vi "send data.vi"() -> ()   [LabVIEW 2016]
uses:
  <vilib>/Instr/_visa.llb/Select Event Type.ctl
  <vilib>/Utility/error.llb/DialogType.ctl
  <vilib>/httpClient/LabVIEWHTTPClient.lvlib
panel:
  in  "Tab Control":enum32{"Page 1", "Page 2"}(tab)
  out "Voltage in range?":bool
  out "Amperage in range?":bool
  out "Pressure in range?":bool
  out "Temperature in range?":bool
  out "Current values":cluster{dbl, dbl, dbl, dbl}(graph)
  in  "VISA resource name":refnum<visa-resource-name>
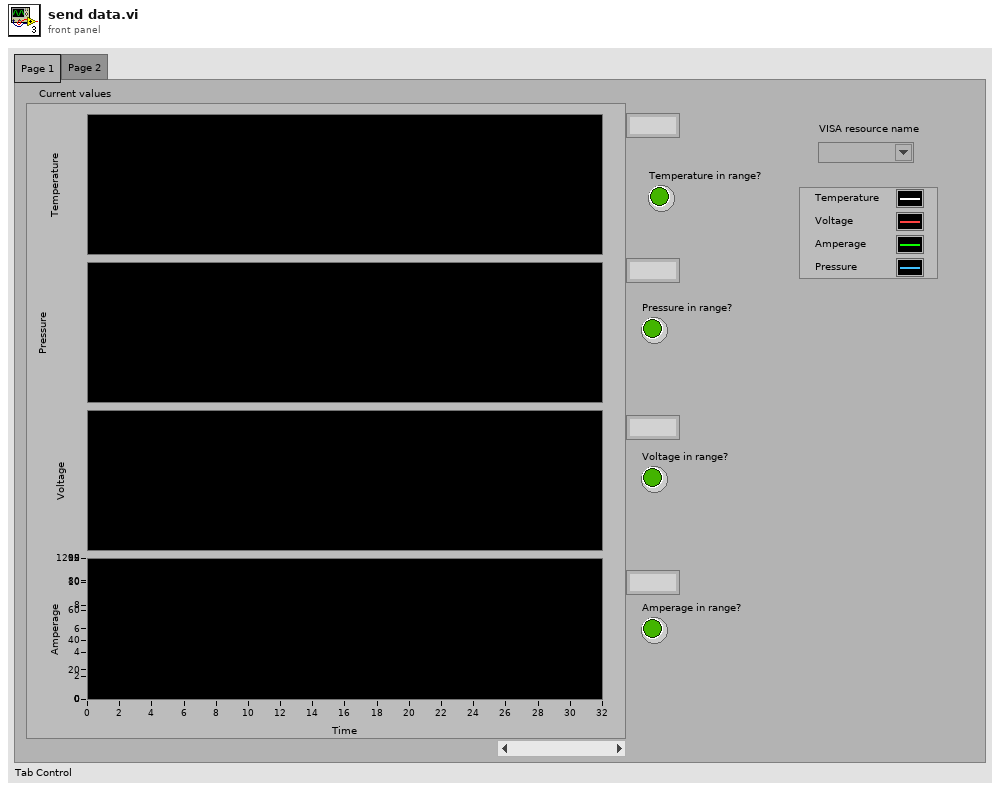
[diagram p1: front panel]
types:
  T1 = typedef "DialogType.ctl" = u16
  T2 = typedef "Select Event Type.ctl" = u32
  T3 = typedef "LabVIEWHTTPClient.lvlib/ClientHandle.ctl" = refnum<k1>
  T4 = cluster{"queue out":refnum<queue>, "queue out":refnum<queue>, "queue out":refnum<queue>, "queue out":refnum<queue>, "queue out":refnum<queue>}
  T5 = cluster{"DS18B20 value":dbl, "BMP180 value":dbl, " potentiometer value":dbl, "ACS712-30A value":dbl}
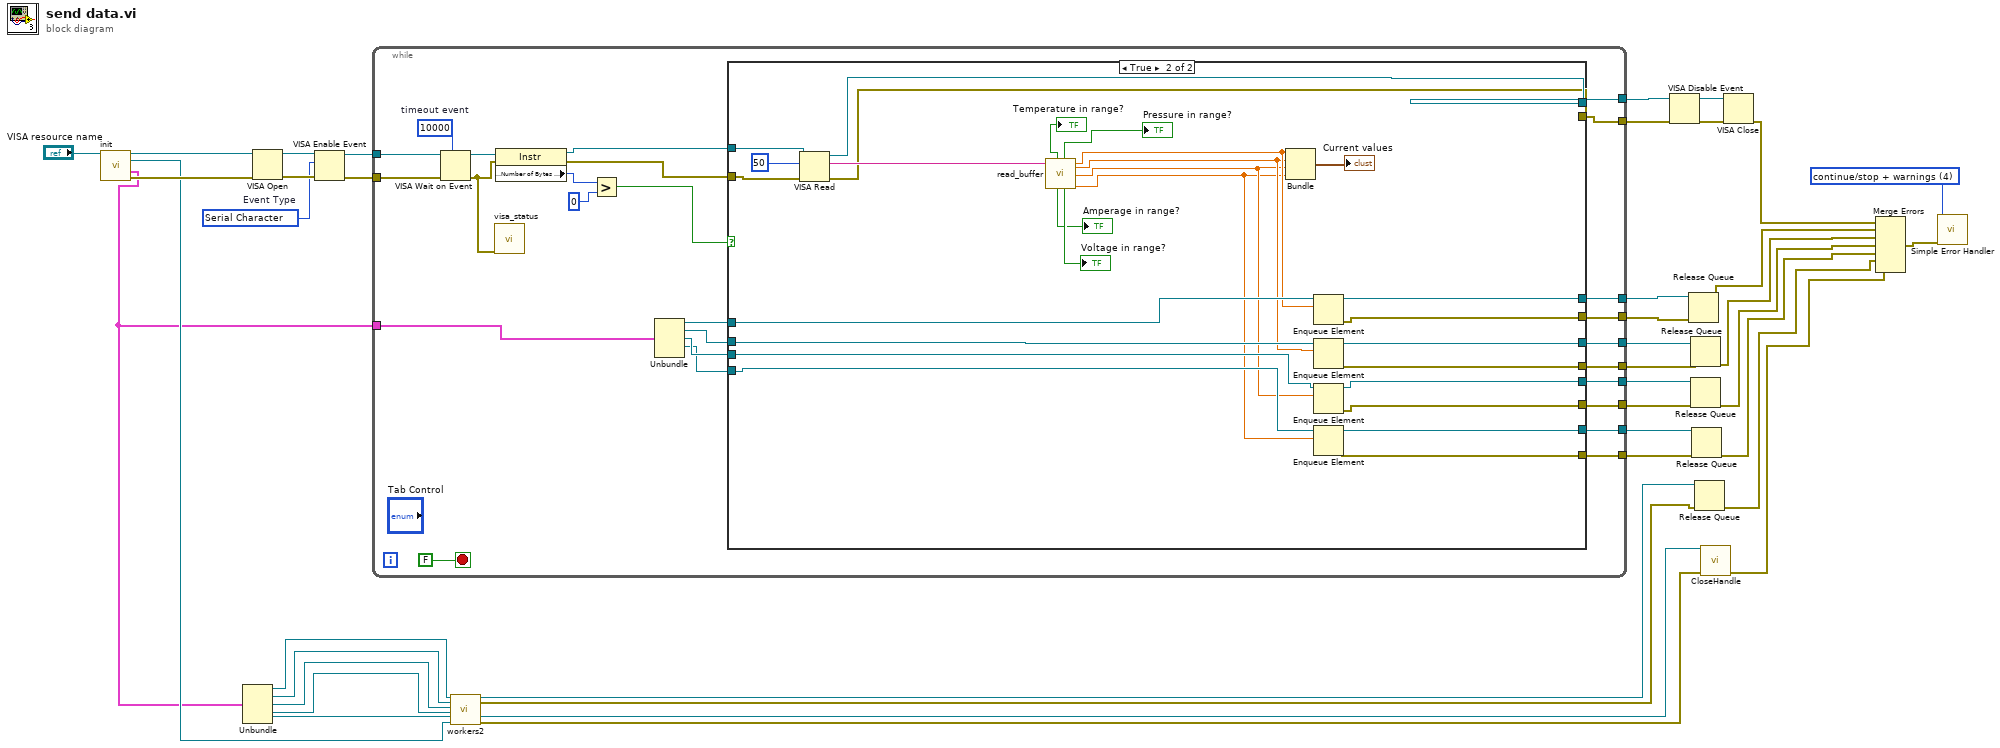
[diagram p0: block diagram]
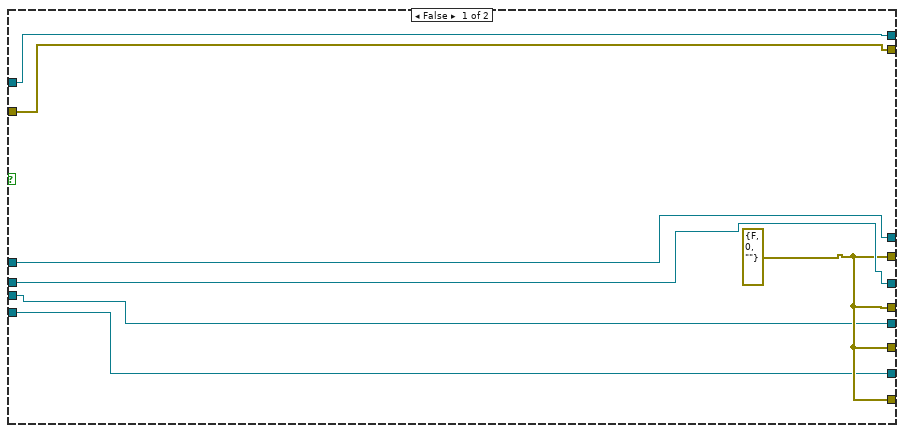
[diagram p2: hidden frame]
diagram:
  w22 = T1 4 items=["no dialog", "OK message", "continue or stop message", "OK message + warnings", "continue/stop + warnings"] ("type of dialog (OK msg:1)")
  w34 = T2 1073684533 items=["Service Request"=1073684491, "Trigger"=3221168138, "Clear"=1073684493, "VXI Signal"=1073684512, "VXI/VME Interrupt"=3221168161, "VXI/VME Sysfail"=1073684509, "VXI/VME Sysreset"=1073684510, "GPIB CIC"=1073684498, "GPIB Talk"=1073684499, "GPIB Listen"=1073684500, "PXI Interrupt"=1073684514, "Serial Break"=1073684515, "Serial TermChar"=1073684516, "Serial CTS"=1073684521, "Serial DSR"=1073684522, "Serial DCD"=1073684524, "Serial RI"=1073684526, "Serial Character"=1073684533, "USB Interrupt"=1073684535, "All Enabled"=1073709055]  # Event Type
  n1 = call "init.vi"("VISA Refnum in"="VISA resource name") -> ("VISA out"=w31:refnum<visa-resource-name>, "client handle out"=w10:T3, "Cluster of queues"=w2:T4, "VISA error out"=w32:errorcluster)  [unwired: 10 in, 1 out]
  n2 = Unbundle(w2) -> ("queue out"=w13:refnum<queue>, "queue out"=w12:refnum<queue>, "queue out"=w11:refnum<queue>, "queue out"=w3:refnum<queue>, "queue out"=w1:refnum<queue>)
  n3 = VISA Open(error in (no error)=w32, VISA resource name=w31) -> (VISA resource name=w40:refnum<visa-resource-name>, error out=w39:errorcluster)  [unwired: 3 in]
  n4 = VISA Enable Event(8:w39, 10:w34, 11:w40) -> (0:w37:errorcluster, 3:w38:refnum<visa-resource-name>)  [unwired: 1 in]
  n5 = while {
    tunnel: w38 -> [w66]
    tunnel: w37 -> [w57]
    tunnel: [w55] -> w30
    tunnel: w2 -> [w54]
    tunnel: [w51] -> w29
    tunnel: [w50] -> w28
    tunnel: [w49] -> w27
    tunnel: [w48] -> w26
    tunnel: [w47] -> w20
    tunnel: [w44] -> w19
    tunnel: [w43] -> w18
    tunnel: [w42] -> w17
    tunnel: [w41] -> w16
    stop <- FALSE stop-if-true
    w59 = u32 10000  # timeout event
    n6 = VISA Wait on Event(7:w59, 8:w57, 11:w66) -> (0:w56:errorcluster, 3:w65:refnum<visa-resource-name>)  [unwired: 2 in, 2 out]
    n7 = call "visa_status.vi"("error in (no error)"=w56) -> ()  [unwired: 11 in]
    n8 = property class="Instr"(reference=w65, error in=w56) -> (reference out=w64:refnum<visa-resource-name>, error out=w60:errorcluster, "Serial Settings:Number of Bytes at Serial Port"=w63:u32)
    n9 = Greater?(x=w63, y=u32 0) -> (0:w61:bool)
    n10 = Unbundle(w54) -> ("queue out"=w53:refnum<queue>, "queue out"=w52:refnum<queue>, "queue out"=w46:refnum<queue>, "queue out"=w45:refnum<queue>)  [unwired: 1 out]
    n11 = case shown="True" w61 {
      tunnel: w64 -> [w72 w99]
      tunnel: w60 -> [w71 w98]
      tunnel: [w72 w92] -> w55
      tunnel: w53 -> [w73 w95]
      tunnel: w52 -> [w70 w96]
      tunnel: [w69 w94] -> w51
      tunnel: [w73 w90] -> w50
      tunnel: [w70 w85] -> w49
      tunnel: [w69 w93] -> w48
      tunnel: [w71 w91] -> w47
      tunnel: w46 -> [w68 w89]
      tunnel: w45 -> [w67 w88]
      tunnel: [w68 w84] -> w44
      tunnel: [w69 w87] -> w43
      tunnel: [w67 w83] -> w42
      tunnel: [w69 w86] -> w41
      frame False {
        w69 = errorcluster {"status"=FALSE, "code"=0, "source"=""} ("error out")
      }
      frame True {
        n12 = VISA Read(VISA resource name=w99, byte count=u32 50, error in (no error)=w98) -> (VISA resource name out=w92:refnum<visa-resource-name>, read buffer=w97:string, error out=w91:errorcluster)  [unwired: 1 out]
        n13 = call "read_buffer.vi"("buffer"=w97) -> ("ACS712-30A value"=w78:dbl, "potentiometer value"=w79:dbl, "BMP180 value"=w80:dbl, "DS18B20 value"=w81:dbl, "Voltage in range?"=→"Voltage in range?":bool, "Pressure in range?"=→"Pressure in range?":bool, "Amperage in range?"=→"Amperage in range?":bool, "Temperature in range?"=→"Temperature in range?":bool)  [unwired: 3 in]
        n14 = Bundle("DS18B20 value"=w81, "BMP180 value"=w80, "potentiometer value"=w79, "ACS712-30A value"=w78) -> (→"Current values":T5)  [unwired: 1 in]
        n15 = Enqueue Element(queue=w95, element=w81) -> (queue out=w90:refnum<queue>, error out=w94:errorcluster)  [unwired: 2 in, 1 out]
        n16 = Enqueue Element(queue=w96, element=w80) -> (queue out=w85:refnum<queue>, error out=w93:errorcluster)  [unwired: 2 in, 1 out]
        n17 = Enqueue Element(queue=w89, element=w79) -> (queue out=w84:refnum<queue>, error out=w87:errorcluster)  [unwired: 2 in, 1 out]
        n18 = Enqueue Element(queue=w88, element=w78) -> (queue out=w83:refnum<queue>, error out=w86:errorcluster)  [unwired: 2 in, 1 out]
      }
    }
  }
  n19 = call "workers2.vi"("queue DS18B20"=w13, "queue BMP180"=w12, "queue potentiometer"=w11, "queue ACS712-30A"=w3, "result queue"=w1, "HTTP client handle"=w10) -> ("result queue out"=w9:refnum<queue>, "result queue error out"=w8:errorcluster, "client handle out"=w6:T3, "client handle error out"=w5:errorcluster)  [unwired: 10 in]
  n20 = VISA Disable Event(8:w20, 11:w30) -> (0:w36:errorcluster, 3:w35:refnum<visa-resource-name>)  [unwired: 2 in]
  n21 = Release Queue(queue=w28, error in (no error)=w29) -> (error out=w24:errorcluster)  [unwired: 1 in, 2 out]
  n22 = Release Queue(queue=w27, error in (no error)=w26) -> (error out=w23:errorcluster)  [unwired: 1 in, 2 out]
  n23 = Release Queue(queue=w19, error in (no error)=w18) -> (error out=w15:errorcluster)  [unwired: 1 in, 2 out]
  n24 = Release Queue(queue=w17, error in (no error)=w16) -> (error out=w14:errorcluster)  [unwired: 1 in, 2 out]
  n25 = Release Queue(queue=w9, error in (no error)=w8) -> (error out=w7:errorcluster)  [unwired: 1 in, 2 out]
  n26 = call <vilib>:"CloseHandle.vi"("client handle"=w6, "error in (no error)"=w5) -> ("error out"=w4:errorcluster)  [unwired: 13 in]
  n27 = VISA Close(VISA resource name=w35, error in (no error)=w36) -> (error out=w25:errorcluster)
  n28 = Merge Errors(w25, w24, w23, w15, w14, w7, w4) -> (w21:errorcluster)
  n29 = call <vilib>:"Simple Error Handler.vi"("type of dialog (OK msg:1)"=w22, "error in (no error)"=w21) -> ()  [unwired: 3 in, 5 out]
